vi "PositionTracer.vi"() -> ()   [LabVIEW 2012]
uses:
  <vilib>/vision/NI_Vision_Development_Module.lvlib
panel:
  in  "Shape Adapted Options in":T1={"Number of Histogram Bins"=8, "Blending Parameter (%)"=10.0, "Max Scale Change (%)"=1.0, "Max Rotation Change"=40.0, "Max Shape Change (%)"=1.0, "Maximum Iterations"=15}
  in  "Pixel size Y":dbl=1.600000023841858
  in  "delay (s)":dbl=-0.9
  out "Y out chart":dbl(graph)
  out "X out chart":dbl(graph)
  out "Any missing frame?":bool
  out "Image":T2(plugin-control)
  in  "Tracking file":path=path "C:/Users/Ludovico/Lavoro/Experiments/Autofocus/vermi/track3.txt"
  in  "Pixel size X":dbl=1.600000023841858
  in  "Interframe time (s)":dbl=0.1
  in  "Image file pattern":string="*tif*"
  in  "Positions file":path=path "C:/Users/Ludovico/Lavoro/Experiments/Autofocus/vermi/CONFSTAGELOG/2016_12_16_10_06.txt"
  in  "Input images folder":path=path "C:/Users/Ludovico/Lavoro/Experiments/Autofocus/vermi/161216_1c_reduced"
  out "error out":errorcluster
  in  "error in (no error)":errorcluster
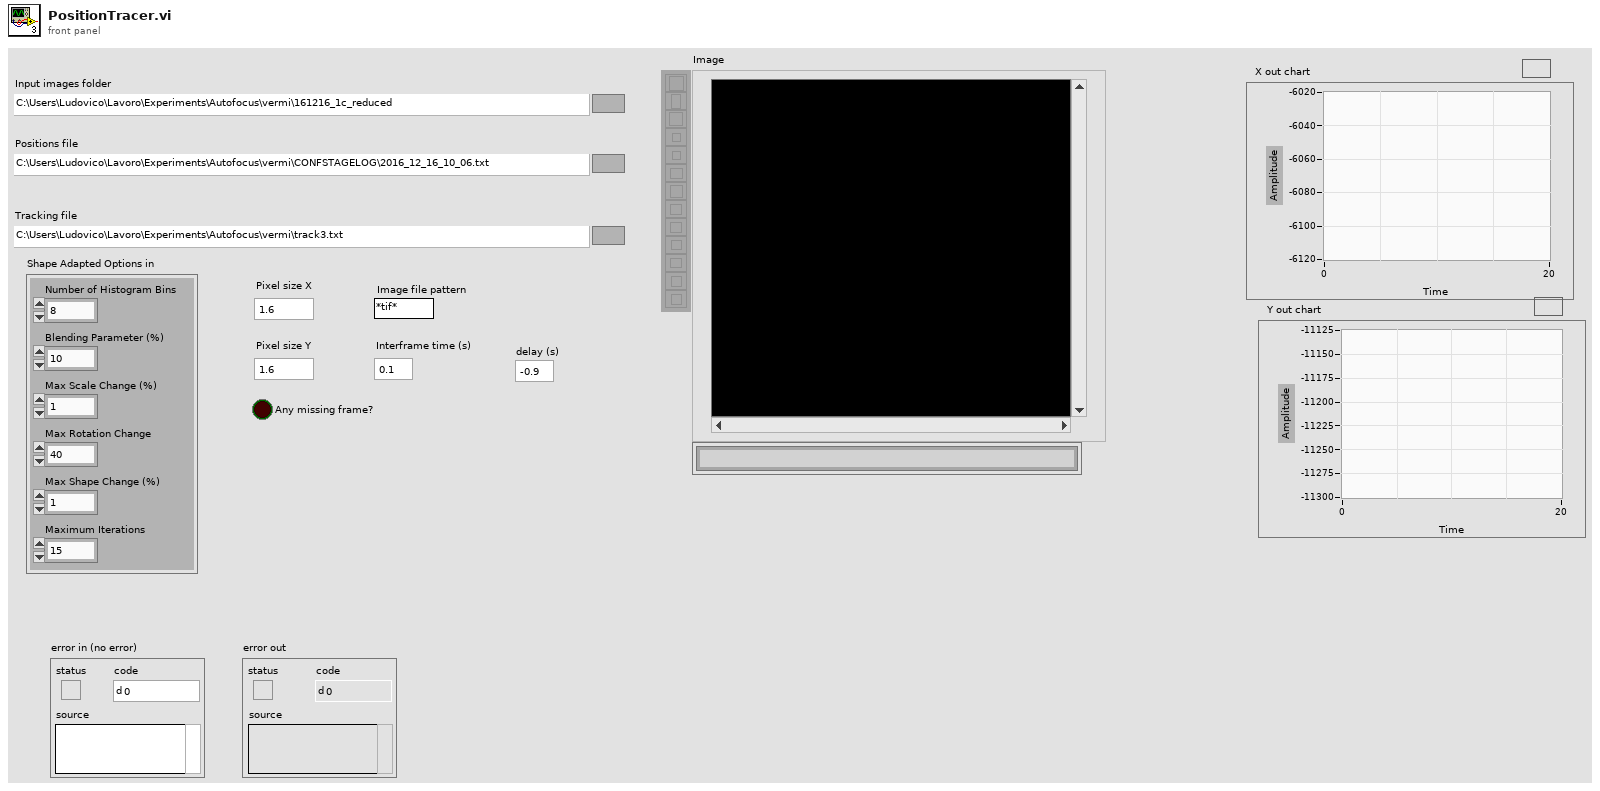
[diagram p1: front panel]
types:
  T1 = cluster{"Number of Histogram Bins":i32, "Blending Parameter (%)":dbl, "Max Scale Change (%)":dbl, "Max Rotation Change":dbl, "Max Shape Change (%)":dbl, "Maximum Iterations":i32}
  T2 = typedef "IMAQ Image.ctl" = refnum<image>
  T3 = cluster{"X":dbl[], "Y":dbl[], "Focus":dbl[], "Time array":dbl[]}
  T4 = typedef "IMAQ Object Tracking Session.ctl" = refnum<k20>
  T5 = typedef "ROI Descriptor" = cluster{"Global Rectangle":i32[], "Contours":cluster{"ID":enum32{"External", "Internal"}, "Type":u32, "Coordinates":i32[]}[]}
  T6 = cluster{"Label":string, "Score":i32, "Angle":dbl, "Location":cluster{"X":dbl, "Y":dbl}, "Bounding Box":cluster{"X":dbl, "Y":dbl}[], "Object Found?":bool}[]
  T7 = cluster{"Label":string, "Score":i32, "Angle":dbl, "Location":cluster{"X":dbl, "Y":dbl}, "Bounding Box":cluster{"X":dbl, "Y":dbl}[], "Object Found?":bool}
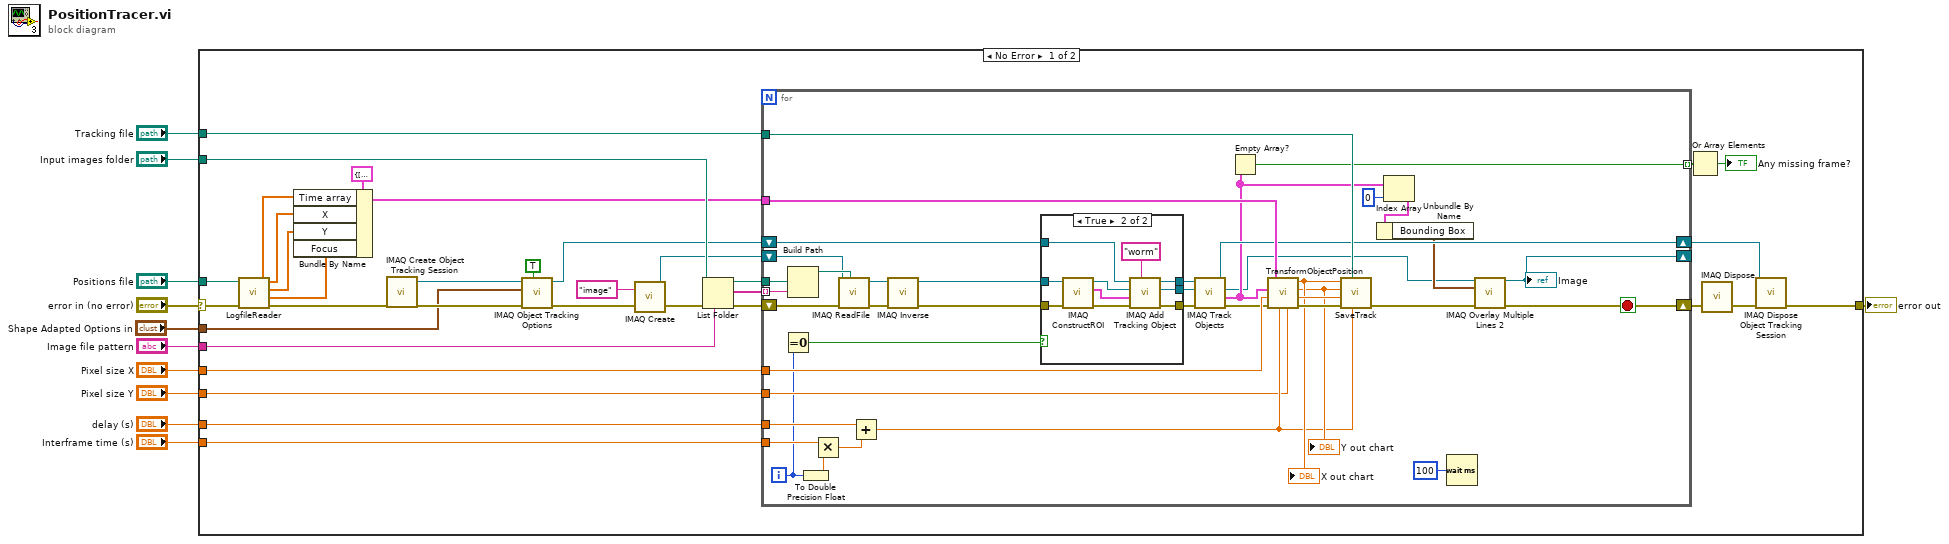
[diagram p0: block diagram]
diagram:
  n1 = case shown="No Error" "error in (no error)" {
    selector: "error in (no error)" -> [w45 w99]
    tunnel: "Positions file" -> [w42 _]
    tunnel: "Input images folder" -> [w41 _]
    tunnel: "Image file pattern" -> [w40 _]
    tunnel: "Interframe time (s)" -> [w29 _]
    tunnel: "Pixel size X" -> [w28 _]
    tunnel: "Tracking file" -> [w27 _]
    tunnel: [w15 w99] -> w4
    tunnel: "delay (s)" -> [w23 _]
    tunnel: "Pixel size Y" -> [w13 _]
    tunnel: "Shape Adapted Options in" -> [w12 _]
    frame No Error {
      n2 = call "LogfileReader.vi"("error in (no error)"=w45, "Positions file"=w42) -> ("error out"=w21:errorcluster, "Focus"=w31:dbl[], "Y"=w32:dbl[], "X"=w33:dbl[], "Time"=w34:dbl[])  [unwired: 5 in]
      n3 = Bundle By Name(cluster=T3 {"X"=[], "Y"=[], "Focus"=[], "Time array"=[]} ("Spacetime cluster"), "Time array"=w34, "X"=w33, "Y"=w32, "Focus"=w31) -> (w30:T3)
      n4 = call "IMAQ Create Object Tracking Session"("error in (no error)"=w21) -> ("error out"=w22:errorcluster, "Object Tracking Session"=w19:T4)  [unwired: 9 in]
      n5 = call-poly "IMAQ Object Tracking Options"("Get/Set (Get)"=TRUE, "error in (no error)"=w22, "Shape Adapted Options in"=w12, "Object Tracking Session In"=w19) -> ("error out"=w20:errorcluster, "Object Tracking Session Out"=w17:T4)  [unwired: 5 in, 1 out]
      n6 = call "IMAQ Create"("Image Name"="image", "error in (no error)"=w20) -> ("New Image"=w36:T2, "error out"=w43:errorcluster)  [unwired: 3 in]
      n7 = List Folder(path=w41, pattern=w40, error in=w43) -> (path out=w37:path, filenames=w38:string[], error out=w39:errorcluster)  [unwired: 1 in, 1 out]
      n8 = for {
        tunnel: w38 -> [w84] mode=indexing
        tunnel: w37 -> [w83]
        shift-right: [w49] -> w26
        shift-left: w39 -> [w85]
        shift-right: [w50] -> _
        shift-left: w36 -> [w81]
        tunnel: w30 -> [w80]
        tunnel: w29 -> [w78]
        tunnel: w28 -> [w77]
        tunnel: w27 -> [w74]
        tunnel: [w72] -> w25 mode=indexing
        tunnel: w23 -> [w68]
        shift-right: [w67] -> w14
        shift-left: w17 -> [w60]
        tunnel: w13 -> [w65]
        i -> [w63]
        stop <- w49 stop-if-true
        n9 = Equal To 0?(x=w63) -> (x = 0?=w62:bool)
        n10 = Build Path(base path=w83, name or relative path=w84) -> (appended path=w82:path)
        n11 = To Double Precision Float(number=w63) -> (double precision float=w79:dbl)
        n12 = Multiply(x=w78, y=w79) -> (x*y=w64:dbl)
        n13 = call "IMAQ ReadFile"("File Path"=w82, "error in (no error)"=w85, "Image"=w81) -> ("error out"=w61:errorcluster, "Image Out"=w48:T2)  [unwired: 4 in, 3 out]
        n14 = Add(x=w68, y=w64) -> (x+y=w69:dbl)
        n15 = call "IMAQ Inverse"("error in (no error)"=w61, "Image Src"=w48) -> ("error out"=w46:errorcluster, "Image Dst Out"=w47:T2)  [unwired: 8 in]
        n16 = case shown="True" w62 {
          tunnel: w47 -> [w88 w98]
          tunnel: w46 -> [w87 w97]
          tunnel: w60 -> [w86 w93]
          tunnel: [w86 w92] -> w59
          tunnel: [w87 w91] -> w58
          tunnel: [w88 w90] -> w57
          frame False {
          }
          frame True {
            n17 = call "IMAQ ConstructROI"("error in (no error)"=w97, "Image"=w98) -> ("error out"=w96:errorcluster, "ROI Descriptor Out"=w94:T5, "Image Out (duplicate)"=w95:T2)  [unwired: 6 in, 1 out]
            n18 = call "IMAQ Add Tracking Object"("Label"="worm", "error in (no error)"=w96, "ROI Descriptor"=w94, "Image"=w95, "Object Tracking Session In"=w93) -> ("error out"=w91:errorcluster, "Image (duplicate)"=w90:T2, "Object Tracking Session Out"=w92:T4)  [unwired: 4 in]
          }
        }
        n19 = call "IMAQ Track Objects"("error in (no error)"=w58, "Image"=w57, "Object Tracking Session In"=w59) -> ("error out"=w66:errorcluster, "Objects (pixel)"=w56:T6, "Image (duplicate)"=w52:T2, "Object Tracking Session Out"=w67:T4)  [unwired: 4 in, 1 out]
        n20 = Empty Array?(array=w56) -> (empty?=w72:bool)
        n21 = call "TransformObjectPosition.vi"("Pixel size Y"=w65, "Image time"=w69, "error in (no error)"=w66, "Pixel size X"=w77, "Objects (pixel)"=w56, "Spacetime cluster"=w80) -> ("error out"=w76:errorcluster, "Focus out"=w75:dbl, "Y out"=w70:dbl, "X out"=w71:dbl)  [unwired: 2 in]
        "X out chart" <- w71
        "Y out chart" <- w70
        n22 = call "SaveTrack.vi"("Time"=w69, "Track file"=w74, "error in (no error)"=w76, "Focus"=w75, "Y"=w70, "X"=w71) -> ("error out"=w51:errorcluster)  [unwired: 5 in]
        n23 = Index Array(array=w56, index=0) -> (element=w54:T7)
        n24 = Unbundle By Name(w54) -> ("Bounding Box"=w53:cluster{"X":dbl, "Y":dbl}[])
        n25 = Wait (ms)(milliseconds to wait=u32 100) -> ()  [unwired: 1 out]
        n26 = call "IMAQ Overlay Multiple Lines 2"("Image"=w52, "Line End Points"=w53, "error in (no error)"=w51) -> ("Image Out"=w50:T2, "error out"=w49:errorcluster)  [unwired: 5 in, 6 out]
        "Image" <- w50
      }
      n27 = Or Array Elements(Boolean array=w25) -> (logical OR=→"Any missing frame?":bool)
      n28 = call "IMAQ Dispose"("error in (no error)"=w26) -> ("error out"=w16:errorcluster)  [unwired: 5 in]
      n29 = call "IMAQ Dispose Object Tracking Session"("error in (no error)"=w16, "Object Tracking Session"=w14) -> ("error out"=w15:errorcluster)  [unwired: 9 in]
    }
    frame Error {
    }
  }
  "error out" <- w4
